vi "Step2.vi"(1 "n":i32, 2 "j":i32, 3 "U":dbl[][](array[numeric]), 4 "X":dbl[][](array[numeric])) -> (0 "v":dbl[](array[numeric]))   [LabVIEW 2011]
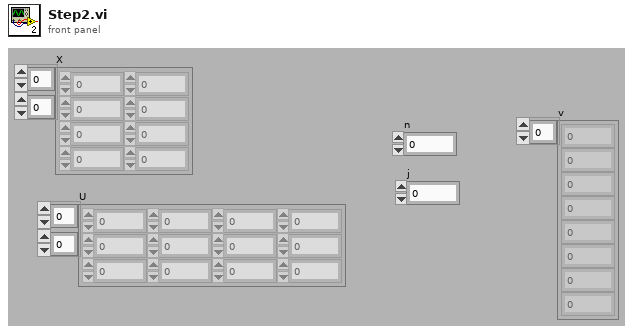
[diagram p1: front panel]
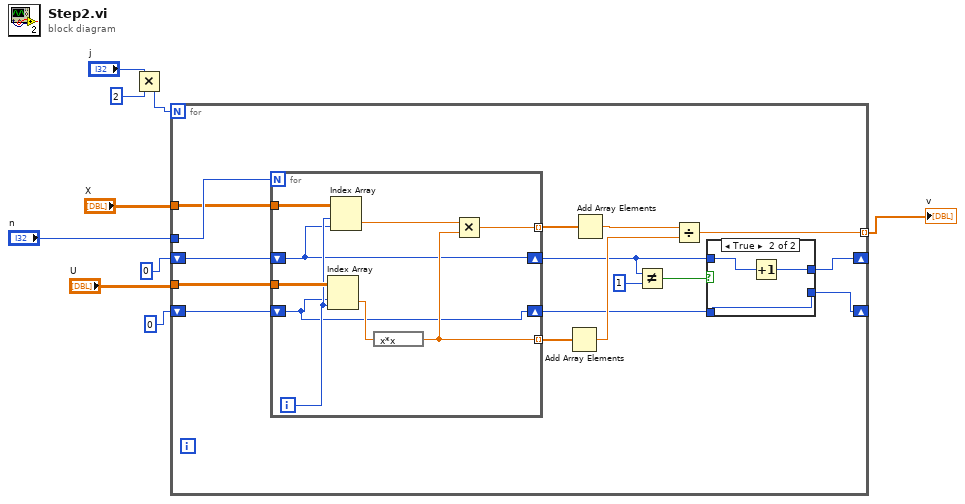
[diagram p0: block diagram]
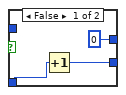
[diagram p2: hidden frame]
diagram:
  n1 = Multiply(x="j", y=2) -> (x*y=w7:i32)
  n2 = for {
    N: w7 -> [_]
    tunnel: "U" -> [w25]
    tunnel: "n" -> [w24]
    tunnel: "X" -> [w22]
    shift-right: [w12] -> _
    shift-left: 0 ("index (row)") -> [w11]
    shift-right: [w19] -> _
    shift-left: 0 ("index (row)") -> [w20]
    tunnel: [w15] -> w5 mode=indexing
    n3 = for {
      N: w24 -> [_]
      tunnel: w25 -> [w40]
      tunnel: [w36] -> w23 mode=indexing
      tunnel: w22 -> [w38]
      tunnel: [w34] -> w21 mode=indexing
      shift-right: [w32] -> w13
      shift-left: w11 -> [w32]
      shift-right: [w33] -> w16
      shift-left: w20 -> [w33]
      i -> [w37]
      n4 = Index Array(array=w40, index (row)=w32, index (col)=w37) -> (element=w39:dbl)
      n5 = Index Array(array=w38, index (row)=w37, index (col)=w33) -> (element=w35:dbl)
      n6 = expression code="x*x"(w39) -> (w36:dbl)
      n7 = Multiply(x=w35, y=w36) -> (x*y=w34:dbl)
    }
    n8 = Add Array Elements(numeric array=w23) -> (sum=w17:dbl)
    n9 = Add Array Elements(numeric array=w21) -> (sum=w18:dbl)
    n10 = Not Equal?(x=w16, y=1) -> (x != y?=w14:bool)
    n11 = Divide(x=w18, y=w17) -> (x/y=w15:dbl)
    n12 = case shown="True" w14 {
      tunnel: w16 -> [_ w31]
      tunnel: [0 w30] -> w19
      tunnel: w13 -> [w27 w29]
      tunnel: [w26 w29] -> w12
      frame False {
        n13 = Increment(x=w27) -> (x+1=w26:i32)
      }
      frame True {
        n14 = Increment(x=w31) -> (x+1=w30:i32)
      }
    }
  }
  "v" <- w5
